vi "Get QueryResponse.vi"(8 "error in (no error)":errorcluster, 11 "gRPCid":T2) -> (0 "error out":errorcluster, 2 "Message Data":T1, 3 "gRPCid out":T2)   [LabVIEW 2016, in "Query Server.lvlib" / "Query Server.lvclass"]
uses:
  Query Server.lvclass
  a51dd2a7-b5c1-4c09-9df4-8cd9d3bd0c19.vi
  QueryResponse_Data.ctl
  gRPC lvSupport/Server API/typeDefs/grpcId.ctl
  gRPC lvSupport/gprc-lvsupport.lvlib
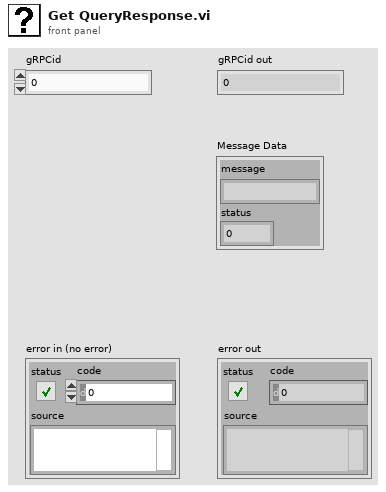
[diagram p1: front panel]
types:
  T1 = typedef "Query Server.lvlib/Query Server.lvclass/QueryResponse_Data.ctl" = cluster{"message":string, "status":i32}
  T2 = typedef "Query Server.lvlib/gprc-lvsupport.lvlib/grpcId.ctl" = u64
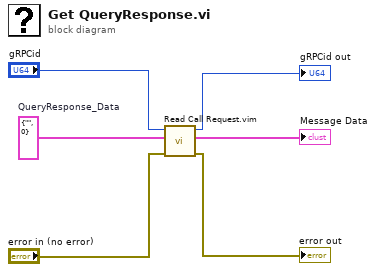
[diagram p0: block diagram]
diagram:
  w2 = T1 {"message"="", "status"=0}  # QueryResponse_Data
  n1 = call "Read Call Request.vim"("error in (no error)"="error in (no error)", "Data Type"=w2, "gRPCid in"="gRPCid") -> ("error out"=→"error out":errorcluster, "Request Data"=→"Message Data":T1, "gRPCid out"=→"gRPCid out":T2)  [unwired: 6 in]
